vi "CAlex2_SetCuff_Pelvis.vi"(8 "Hip Cuff Forward Shift":dbl, 9 "Hip Cuff Height":dbl, 10 "Hip Cuff Width":dbl, 11 "Hip Width":dbl) -> (3 "Hip Cuff":T1={"BodyID"=0, "CoM(CuffCS)"={"Coord4"=[0.0, 0.0, 0.0, 1.0], "ID"=0}, "Mass(kg)"=0.0, "CablePts(CuffCS)"=[], "Cuff->Body"=[[1.0, 0.0, 0.0, 0.0], [0.0, 1.0, 0.0, 0.0], [0.0, 0.0, 1.0, 0.0], [0.0, 0.0, 0.0, 1.0]]})   [LabVIEW 2015, in "CAlex2.lvclass"]
uses:
  CAlex2.lvclass
  CableSerialChain/TypeDef/Cuff.ctl
  Body/PointOnBody.ctl
  <vilib>/Analysis/Matrix/Datatypes/RealMatrix.ctl
  Body/xyzO.ctl
  Body/Bodies.lvclass
  <vilib>/Analysis/Matrix/NI_Matrix.lvlib
  CableSerialChain/CableSerialChain.lvclass
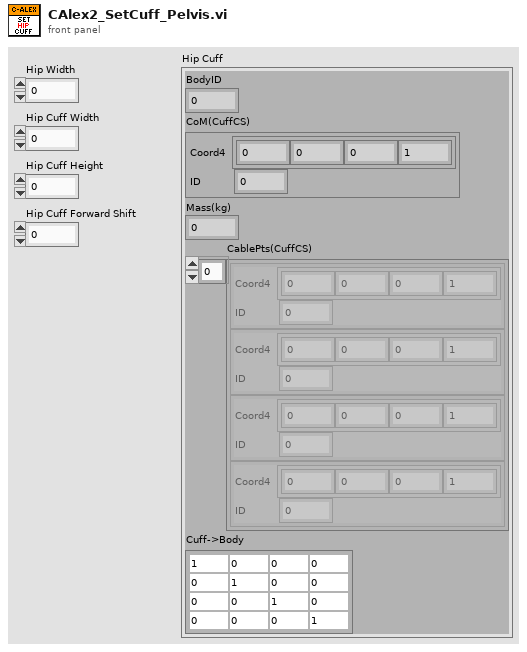
[diagram p1: front panel]
types:
  T1 = typedef "CableSerialChain.lvclass/Cuff.ctl" = cluster{"BodyID":i32, "CoM(CuffCS)":T2, "Mass(kg)":dbl, "CablePts(CuffCS)":T2[], "Cuff->Body":T3}
  T2 = typedef "Bodies.lvclass/PointOnBody.ctl" = cluster{"Coord4":dbl[], "ID":i32}
  T3 = typedef "NI_Matrix.lvlib/RealMatrix.ctl" = dbl[][]
  T4 = typedef "Bodies.lvclass/xyzO.ctl" = enum16{"X", "Y", "Z", "O"}
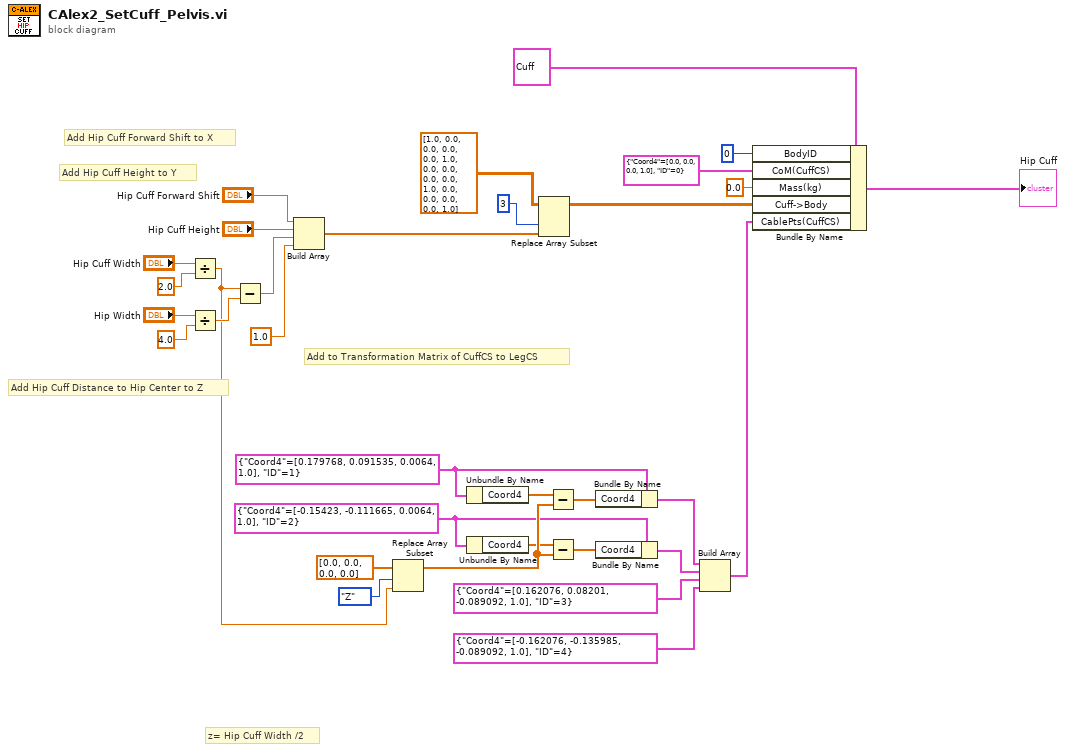
[diagram p0: block diagram]
diagram:
  w2 = T2 {"Coord4"=[0.179768, 0.091535, 0.0064, 1.0], "ID"=1} ("CoM(CuffCS)")
  w1 = T2 {"Coord4"=[-0.15423, -0.111665, 0.0064, 1.0], "ID"=2} ("CoM(CuffCS)")
  # "Add to Transformation Matrix of CuffCS to LegCS"
  # "Add Hip Cuff Distance to Hip Center to Z"
  # "Add Hip Cuff Forward Shift to X"
  # "z= Hip Cuff Width /2"
  # "Add Hip Cuff Height to Y"
  n1 = Divide(x="Hip Cuff Width", y=2.0) -> (x/y=w10:dbl)
  n2 = Divide(x="Hip Width", y=4.0) -> (x/y=w11:dbl)
  n3 = Subtract(x=w10, y=w11) -> (x-y=w9:dbl)
  n4 = Build Array("Hip Cuff Forward Shift", "Hip Cuff Height", w9, 1.0 ("BodyNum")) -> (w5:dbl[])
  n5 = Replace Array Subset(array=dbl[] [0.0, 0.0, 0.0, 0.0] ("Coord4"), new element=w10, index=xyzO."Z" ("XYZ")) -> (w25:dbl[])
  n6 = Unbundle By Name(w2) -> ("Coord4"=w21:dbl[])
  n7 = Unbundle By Name(w1) -> ("Coord4"=w24:dbl[])
  n8 = Replace Array Subset(array=T3 [[1.0, 0.0, 0.0, 0.0], [0.0, 1.0, 0.0, 0.0], [0.0, 0.0, 1.0, 0.0], [0.0, 0.0, 0.0, 1.0]] ("Cuff->Leg"), new element=w5, index (col)=3 ("index (row)")) -> (w28:T3)  [unwired: 1 in]
  n9 = Subtract(x=w21, y=w25) -> (x-y=w26:dbl[])
  n10 = Subtract(x=w24, y=w25) -> (x-y=w27:dbl[])
  n11 = Bundle By Name(cluster=w2, "Coord4"=w26) -> (w17:T2)
  n12 = Bundle By Name(cluster=w1, "Coord4"=w27) -> (w18:T2)
  n13 = Build Array(w17, w18, T2 {"Coord4"=[0.162076, 0.08201, -0.089092, 1.0], "ID"=3} ("CoM(CuffCS)"), T2 {"Coord4"=[-0.162076, -0.135985, -0.089092, 1.0], "ID"=4} ("CoM(CuffCS)")) -> (w16:T2[])
  n14 = Bundle By Name(cluster=T1 {"BodyID"=0, "CoM(CuffCS)"={"Coord4"=[0.0, 0.0, 0.0, 1.0], "ID"=0}, "Mass(kg)"=0.0, "CablePts(CuffCS)"=[], "Cuff->Body"=[[1.0, 0.0, 0.0, 0.0], [0.0, 1.0, 0.0, 0.0], [0.0, 0.0, 1.0, 0.0], [0.0, 0.0, 0.0, 1.0]]} ("Cuff Design"), "BodyID"=0, "CoM(CuffCS)"=T2 {"Coord4"=[0.0, 0.0, 0.0, 1.0], "ID"=0}, "Mass(kg)"=0.0, "Cuff->Body"=w28, "CablePts(CuffCS)"=w16) -> (→"Hip Cuff":T1)
